vi "Untitled 1.vi"() -> ()   [LabVIEW 2015]
uses:
  <vilib>/httpClient/LabVIEWHTTPClient.lvlib
panel:
  out "Cluster":cluster{"headers":string, "body":string}
  in  "Enum":T1(ring)
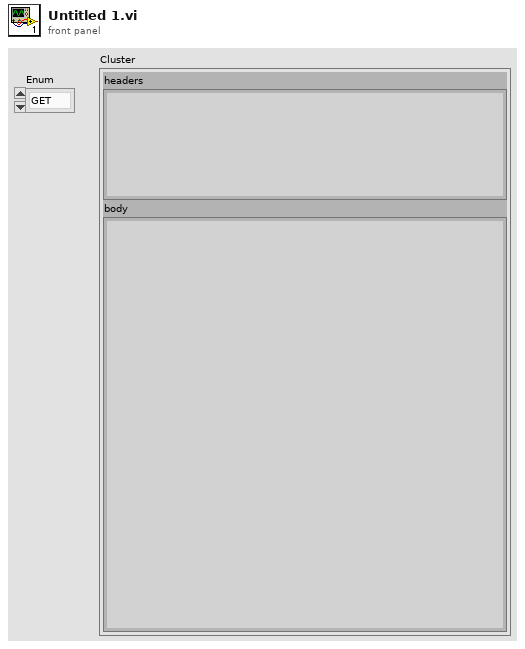
[diagram p1: front panel]
types:
  T1 = enum16{"GET", "POST", "PUT", "DELETE", "UPDATE", "EXIT"}
  T2 = typedef "LabVIEWHTTPClient.lvlib/ClientHandle.ctl" = refnum<k1>
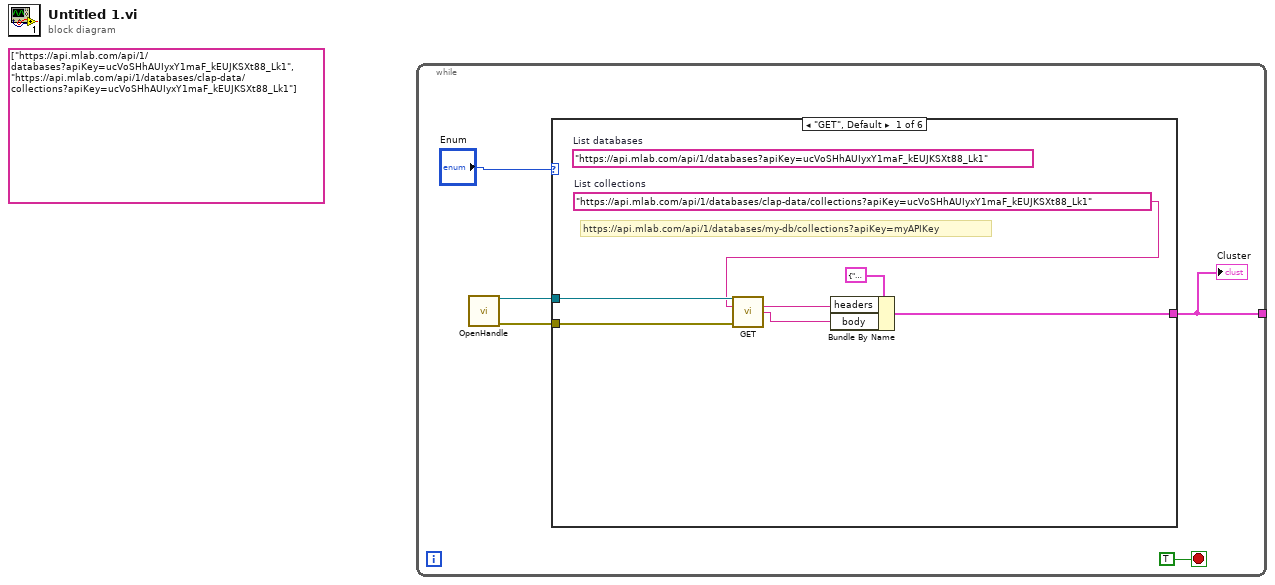
[diagram p0: block diagram]
diagram:
  (unwired) string[] ["https://api.mlab.com/api/1/databases?apiKey=ucVoSHhAUIyxY1maF_kEUJKSXt88_Lk1", "https://api.mlab.com/api/1/databases/clap-data/collections?apiKey=ucVoSHhAUIyxY1maF_kEUJKSXt88_Lk1"]
  n1 = while {
    tunnel: [w4] -> _
    stop <- TRUE stop-if-true
    n2 = call <vilib>:"OpenHandle.vi"() -> ("client handle out"=w3:T2, "error out"=w2:errorcluster)  [unwired: 14 in]
    n3 = case shown="\"GET\", Default" "Enum" {
      tunnel: [w9 _ _ _ _ _] -> w4
      tunnel: w3 -> [w8 _ _ _ _ _]
      tunnel: w2 -> [w7 _ _ _ _ _]
      frame "GET", Default {
        w6 = "https://api.mlab.com/api/1/databases/clap-data/collections?apiKey=ucVoSHhAUIyxY1maF_kEUJKSXt88_Lk1"  # List collections
        (unwired) "https://api.mlab.com/api/1/databases?apiKey=ucVoSHhAUIyxY1maF_kEUJKSXt88_Lk1"  # List databases
        # "https://api.mlab.com/api/1/databases/my-db/collections?apiKey=myAPIKey"
        n4 = call <vilib>:"GET.vi"("client handle"=w8, "url"=w6, "error in (no error)"=w7) -> ("headers"=w11:string, "body"=w10:string)  [unwired: 9 in, 2 out]
        n5 = Bundle By Name(cluster=cluster{"headers":string, "body":string} {"headers"="", "body"=""}, "headers"=w11, "body"=w10) -> (w9:cluster{"headers":string, "body":string})
      }
      frame "POST" {
      }
      frame "PUT" {
      }
      frame "DELETE" {
      }
      frame "UPDATE" {
      }
      frame "EXIT" {
      }
    }
    "Cluster" <- w4
  }
